vi "myRIO_BRig_RT__Case_Exp_State_Selection.vi"(0 "input_dataCurrent":u16[](array[numeric]), 1 "input_dataExp":u16[](array[numeric]), 3 "input_state":T1, 4 "input_spout":enum16{"Left", "Right"}(ring), 8 "I_lick":bool, 10 "I_lick_left":bool) -> (14 "output_dataCurrent":u16[](array[numeric]), 17 "output_state":T1)   [LabVIEW 2014]
uses:
  myRIO_BRig_RT__Case_Exp_stateList.ctl
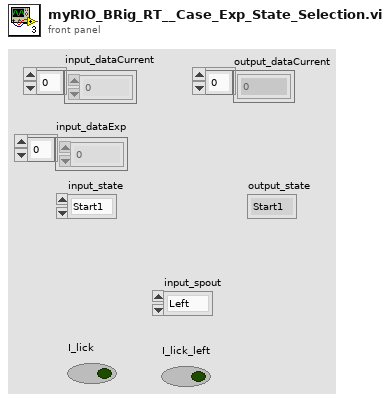
[diagram p1: front panel]
types:
  T1 = typedef "myRIO_BRig_RT__Case_Exp_stateList.ctl" = enum16{"Start1", "Start2", "Start3", "saveSettings1", "saveSettings2", "saveSettings3", "saveSettings4_LC_ENL", "saveSettings5_LC_Cue", "saveSettings6_LC_Other", "setSettings_Audio", "initBlock_pre", "initBlock", "initBlock2", "initBlock_post", "initTrial_pre", "initTrial", "initTrial2", "initTrial_post", "ENL1_pre", "ENL1", "ENL1_post", "ENL1Penalty_pre", "ENL1Penalty", "ENL2_pre", "ENL2", "ENL2Penalty_pre", "ENL2Penalty", "Cue1_pre", "Cue1", "Cue1_post", "Cue1Penalty_pre", "Cue1Penalty", "Cue2_pre", "Cue2", "Cue2Penalty_pre", "Cue2Penalty", "Selection_pre", "Selection", "Select_post", "SelectReward_pre", "SelectReward", "SelectRewardPost_pre", "SelectRewardPost", "SelectWrong_pre", "SelectWrong", "SelectWrong_post", "SelectTimeout_pre", "SelectTimeout", "SelectTimeout_post", "endTrial_pre", "endTrial1", "endTrial2", "endTrial3", "endTrial_post", "endBlock_pre", "endBlock", "endBlock_post", "endExp", "commConnect", "commUpload_pre", "commUpload_dataBlock", "commUpload_dataCurrent", "commUpload_dataExp", "commUpload_dataLC", "commUpload_dataTrial", "commUpload_post", "saveData_pre", "saveData_dataBlock", "saveData_dataCurrent", "saveData_dataExp", "saveData_dataLC", "saveData_dataTrial", "saveData_post"}
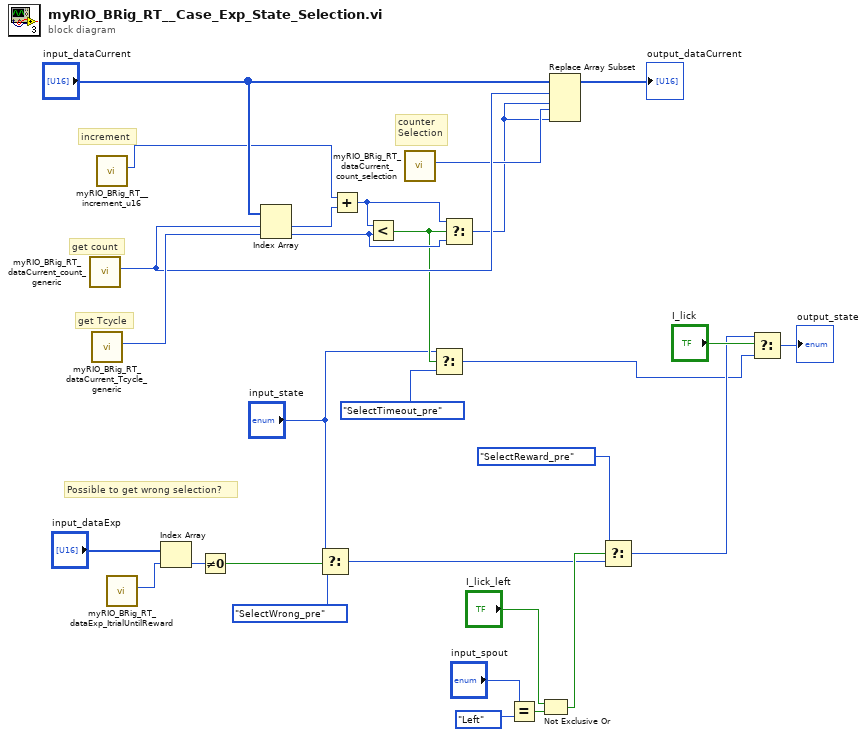
[diagram p0: block diagram]
diagram:
  # "counter\nSelection"
  # "increment"
  # "Possible to get wrong selection?"
  # "get Tcycle"
  # "get count"
  n1 = call "myRIO_BRig_RT_dataCurrent_count_generic.vi"() -> ("output_count_generic"=w25:i32)  [unwired: 11 in]
  n2 = call "myRIO_BRig_RT_dataCurrent_Tcycle_generic.vi"() -> ("output_Tcycle_generic"=w27:i32)  [unwired: 11 in]
  n3 = call "myRIO_BRig_RT__increment_u16.vi"() -> ("output_increment__u16"=w9:u16)  [unwired: 11 in]
  n4 = call "myRIO_BRig_RT_dataExp_ItrialUntilReward.vi"() -> ("output_I_trialUntilReward"=w20:i32)  [unwired: 11 in]
  n5 = Index Array(array="input_dataExp", index=w20) -> (element=w19:u16)
  n6 = Not Equal To 0?(x=w19) -> (x != 0?=w18:bool)
  n7 = Index Array(array="input_dataCurrent", index #1=w25, index #2=w27) -> (element #1=w26:u16, element #2=w24:u16)
  n8 = Select(t="input_state", s=w18, f=myRIO_BRig_RT__Case_Exp_stateList."SelectWrong_pre" ("Enum")) -> (s? t:f=w14:T1)
  n9 = Add(x=w9, y=w26) -> (x+y=w2:u16)
  n10 = Less?(x=w2, y=w24) -> (x < y?=w11:bool)
  n11 = call "myRIO_BRig_RT_dataCurrent_count_selection.vi"() -> ("output_count_generic"=w3:i32)  [unwired: 11 in]
  n12 = Select(t="input_state", s=w11, f=myRIO_BRig_RT__Case_Exp_stateList."SelectTimeout_pre" ("Enum")) -> (s? t:f=w10:T1)
  n13 = Select(t=w2, s=w11, f=w24) -> (s? t:f=w1:u16)
  n14 = Equal?(x="input_spout", y=enum16{"Left", "Right"}."Left") -> (x = y?=w17:bool)
  n15 = Not Exclusive Or(1:w17, 2:"I_lick_left") -> (0:w15:bool)
  n16 = Replace Array Subset(array="input_dataCurrent", new element #1=w1, index #1=w25, new element #2=w1, index #2=w3) -> (→"output_dataCurrent":u16[])
  n17 = Select(t=myRIO_BRig_RT__Case_Exp_stateList."SelectReward_pre" ("Enum"), s=w15, f=w14) -> (s? t:f=w12:T1)
  n18 = Select(t=w12, s="I_lick", f=w10) -> (s? t:f=→"output_state":T1)
